vi "CAEN_HVSystem.EUString2UnitMultilier.vi"(3 "error in (no error)":errorcluster, 5 "EU String":string) -> (0 "error out":errorcluster, 1 "Multiplier":dbl format="%#.1e", 2 "Unit":string)   [LabVIEW 2014, in "CAEN_HVSystem.lvlib"]
doc: "This VI converts the EU string to Unit string and Multiplier.\n\nHere is our list of EU strings:\n\n\"Volt\" for the voltage items\n\"Watt\" for the power items\n\"Celsius\" for temperature items\n\"Amp.\" for the current items\n\"Hz\" for the frequency items\n\"Bar\" for pressure items\n\"Volt/sec\" for Ramp/Up Ramp/Down items\n\"Sec.\" for the time items\n\"rpm\" for the fan items\n\"count\" to represent a binary value\n\"None\" for scalar items\n\nfor each list we associate the followinf scale:\n\n\"K\" for KILO\n\"M\" for MEGA\n\"G\" for GIGA\n\"T\" for TERA\n\"m\" for MILLI\n\"u\" for MICRO\n\"n\" for NANO\n\"p\" for PICO\n\"\" elsewhere\n\nThe units (EU Strings) are constant so i.e. if an item is represented as a uAmp it's scale will be always represented as uAmp for each values it can returns ( t0= 10 uAmp t1=10000 uAmp).\n\nBest Regards,\nAlberto Dimaio, CAEN"
uses:
  CAEN_HVSystem.lvlib
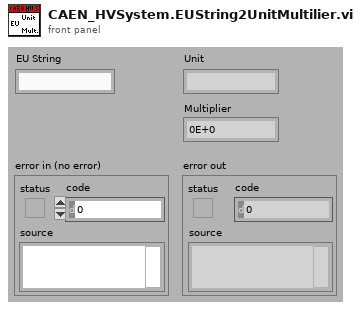
[diagram p1: front panel]
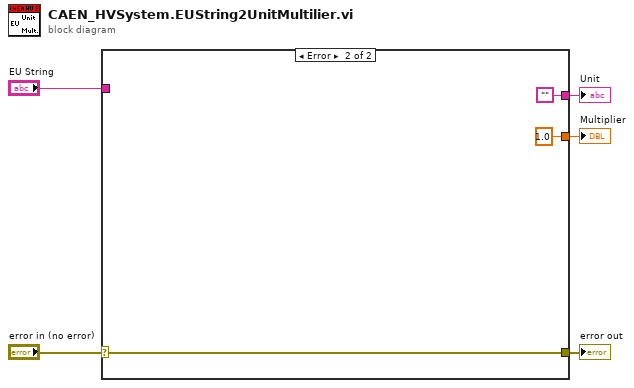
[diagram p0: block diagram]
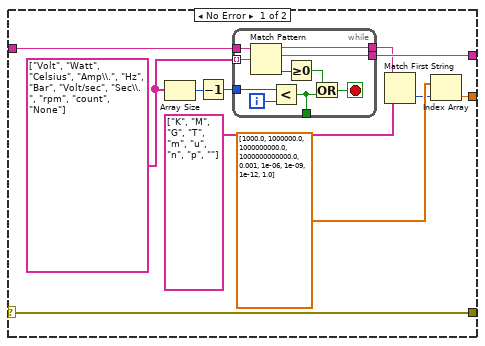
[diagram p2: hidden frame]
diagram:
  n1 = case shown="Error" "error in (no error)" {
    selector: "error in (no error)" -> [w6 w29]
    tunnel: "EU String" -> [w16 _]
    tunnel: [w14 ""] -> w4
    tunnel: [w12 1.0] -> w3
    tunnel: [w6 w29] -> w1
    frame No Error {
      w15 = string[] ["Volt", "Watt", "Celsius", "Amp\\.", "Hz", "Bar", "Volt/sec", "Sec\\.", "rpm", "count", "None"]
      n2 = Array Size(array=w15) -> (size(s)=w8:i32)
      n3 = Decrement(x=w8) -> (x-1=w7:i32)
      n4 = while {
        tunnel: w16 -> [w26]
        tunnel: w15 -> [w25] mode=indexing
        tunnel: [w24] -> w9
        tunnel: [w23] -> w14
        tunnel: w7 -> [w20]
        tunnel: [w17] -> _
        i -> [w21]
        stop <- w18 stop-if-true
        n5 = Match Pattern(string=w26, regular expression=w25) -> (before substring=w24:string, match substring=w23:string, offset past match=w22:i32)  [unwired: 1 in, 1 out]
        n6 = Less?(x=w20, y=w21) -> (x < y?=w17:bool)
        n7 = Greater Or Equal To 0?(x=w22) -> (x >= 0?=w19:bool)
        n8 = Or(x=w19, y=w17) -> (x .or. y?=w18:bool)
      }
      n9 = Match First String(2:string[] ["K", "M", "G", "T", "m", "u", "n", "p", ""], 3:w9) -> (0:w10:i32)  [unwired: 1 out]
      n10 = Index Array(array=dbl[] [1000.0, 1000000.0, 1000000000.0, 1000000000000.0, 0.001, 1e-06, 1e-09, 1e-12, 1.0], index=w10) -> (element=w12:dbl)
    }
    frame Error {
    }
  }
  "Unit" <- w4
  "Multiplier" <- w3
  "error out" <- w1
